vi "Seq Get Current Sequence.vi"(6 "config paths":T1, 8 "Error In":errorcluster, 9 "Segment Info In":T2, 10 "Basic Steps":string[](array[string]), 11 "VI Names":string[](array[string])) -> (0 "Error Out":errorcluster, 2 "Step Hisitory":string[](array[string]))   [LabVIEW 2018]
uses:
  type defs/Sequence Info.ctl
  type defs/config paths for seq def.ctl
panel:
  out "appended path":path
  out "file or folder exists?":bool
  out "File Name":string
  out "Add Step?":bool
  out "Segment Info Out":T2
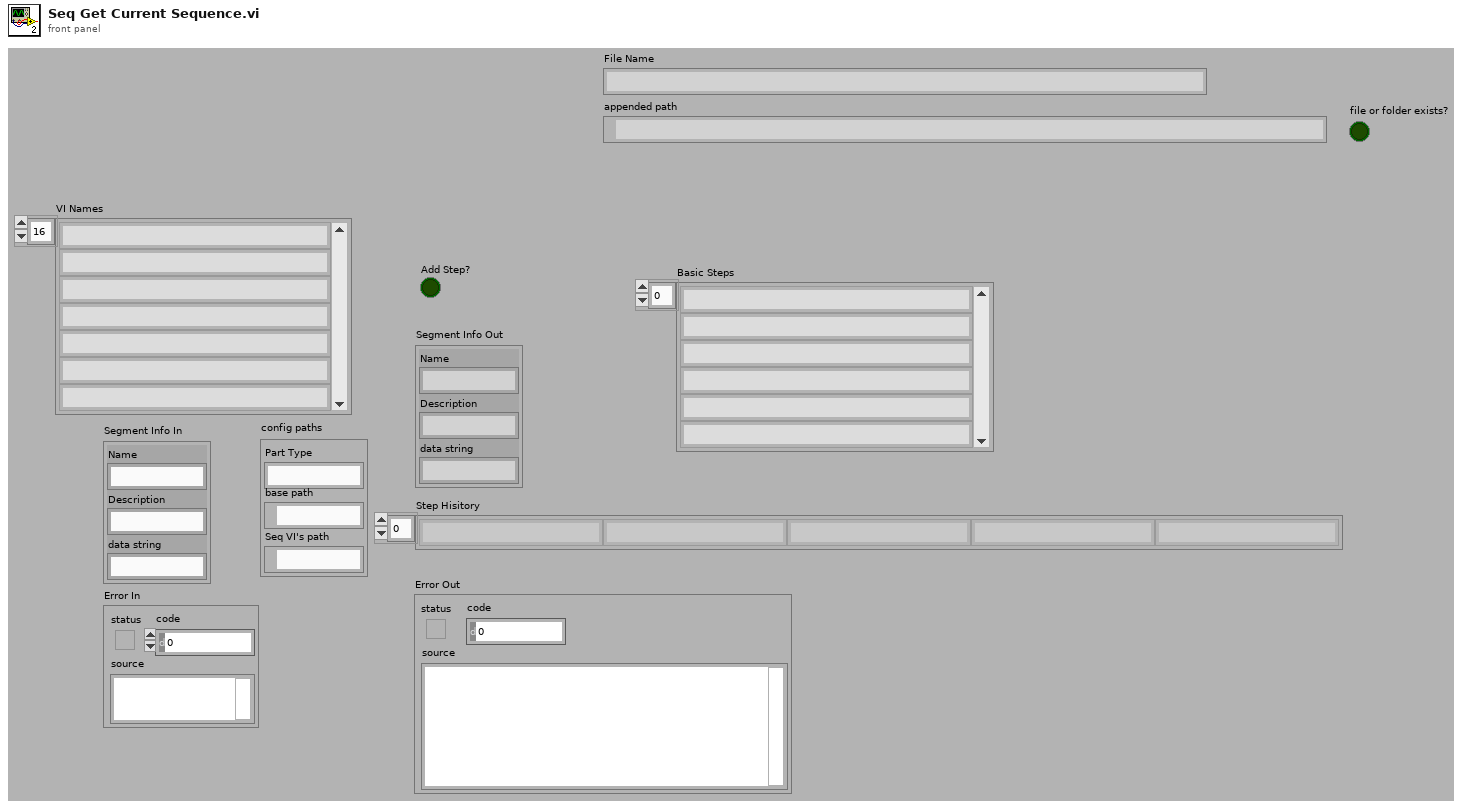
[diagram p1: front panel]
types:
  T1 = typedef "config paths for seq def.ctl" = cluster{"Part Type":string, "base path":path, "Seq VI's path":path}
  T2 = typedef "Sequence Info.ctl" = cluster{"Name":string, "Description":string, "data string":string}
  T3 = enum32{"Bad", "Idle", "Run top level", "Running"}
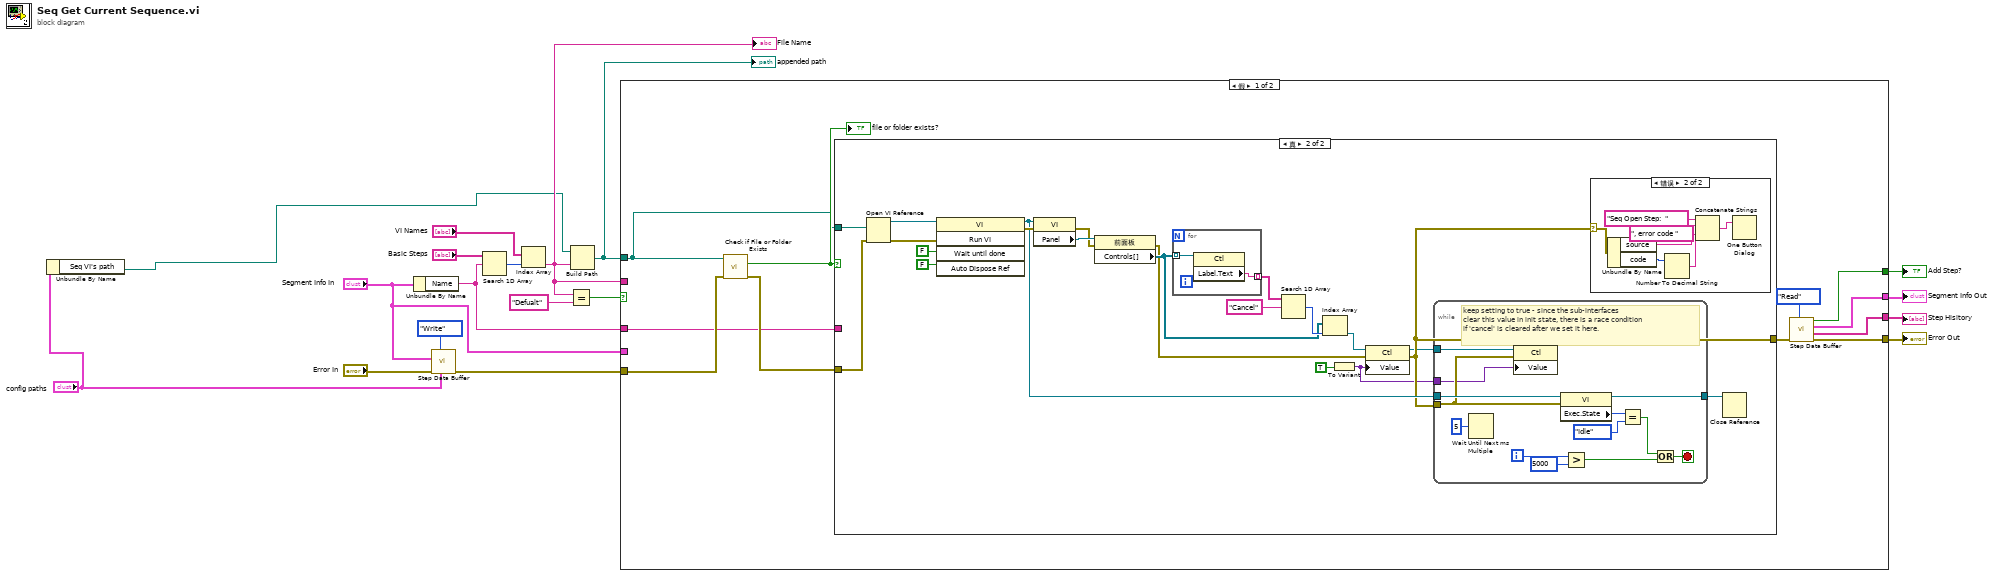
[diagram p0: block diagram]
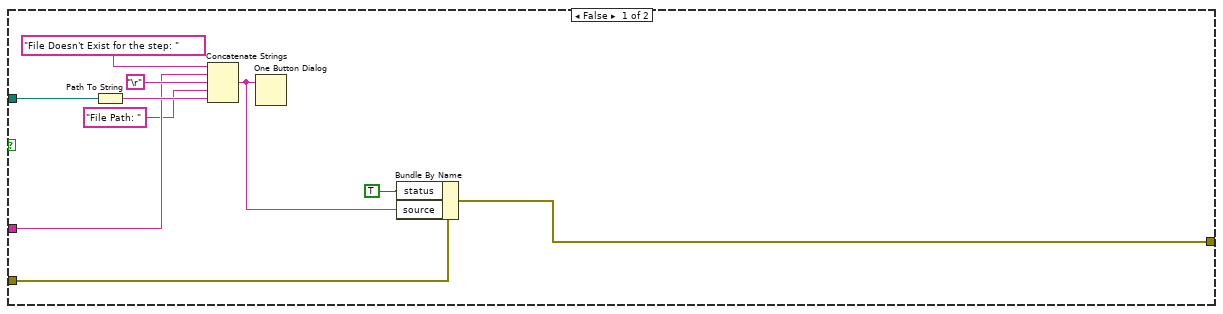
[diagram p2: hidden frame]
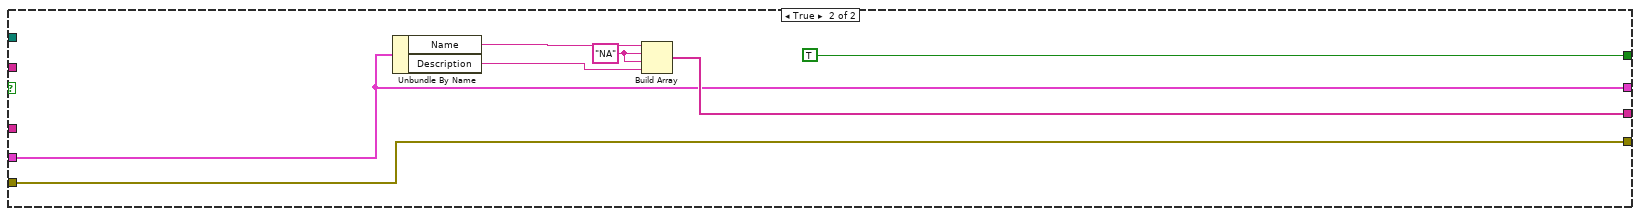
[diagram p4: hidden frame]
diagram:
  n1 = Unbundle By Name("config paths") -> ("Seq VI's path"=w1:path)
  n2 = Unbundle By Name("Segment Info In") -> ("Name"=w14:string)
  n3 = call "Step Data Buffer.vi"("config paths"="config paths", "Mode"=enum16{"Init", "Read", "Write"}."Write", "Error In"="Error In", "Segment Data"="Segment Info In") -> ("Error Out"=w11:errorcluster)  [unwired: 3 in, 4 out]
  n4 = Search 1D Array(1D array="Basic Steps", element=w14) -> (index of element=w10:i32)  [unwired: 1 in]
  n5 = Index Array(array="VI Names", index=w10) -> (element=w3:string)
  "File Name" <- w3
  n6 = Equal?(x=w3, y="Defualt") -> (x = y?=w8:bool)
  n7 = Build Path(base path=w1, name or relative path=w3) -> (appended path=w7:path)
  "appended path" <- w7
  n8 = case shown="假" w8 {
    tunnel: w7 -> [w28 _]
    tunnel: w11 -> [w27 w87]
    tunnel: [w23 w87] -> w15
    tunnel: w14 -> [w19 _]
    tunnel: [w22 w88] -> w18
    tunnel: [w20 TRUE ("Add Step?")] -> w6
    tunnel: "Segment Info In" -> [_ w85]
    tunnel: [w21 w85] -> w4
    tunnel: w3 -> [_ _]
    frame False {
      n9 = call <vilib>:"Check if File or Folder Exists.vi"("error in (no error)"=w27, "path"=w28) -> ("error out"=w26:errorcluster, "file or folder exists?"=w29:bool)  [unwired: 7 in, 1 out]
      "file or folder exists?" <- w29
      n10 = case shown="真" w29 {
        tunnel: w28 -> [w39 w60]
        tunnel: [w32 w46] -> w24
        tunnel: w26 -> [w33 w59]
        tunnel: w19 -> [w35 _]
        frame False {
          n11 = Path To String(path=w39) -> (string=w38:string)
          n12 = Concatenate Strings("File Doesn't Exist for the step: " ("string"), w35, "\r", "File Path: " ("string"), w38) -> (w31:string)
          n13 = One Button Dialog(message=w31) -> ()  [unwired: 1 in, 1 out]
          n14 = Bundle By Name(cluster=w33, "status"=TRUE, "source"=w31) -> (w32:errorcluster)
        }
        frame True {
          n15 = Open VI Reference(vi path=w60, error in (no error)=w59) -> (vi reference=w43:refnum<vi>, error out=w44:errorcluster)  [unwired: 4 in]
          n16 = invoke class="VI" method="Run VI"(reference=w43, error in=w44, "Wait until done"=FALSE ("Wait Until Done"), "Auto Dispose Ref"=FALSE ("Auto Dispose Reference")) -> (reference out=w47:refnum<vi>, error out=w49:errorcluster)  [unwired: 1 in, 3 out]
          n17 = property class="VI"(reference=w47, error in=w49) -> (error out=w50:errorcluster, "Panel"=w57:refnum<vi>)  [unwired: 1 out]
          n18 = property class="前面板"(reference=w57, error in=w50) -> (error out=w42:errorcluster, "Controls[]"=w53:refnum<vi>[])  [unwired: 1 out]
          n19 = for {
            tunnel: w53 -> [w75] mode=indexing
            tunnel: [w74] -> w56 mode=indexing
            n20 = property class="Ctl"(reference=w75) -> ("Label.Text"=w74:string)  [unwired: 1 in, 2 out]
          }
          n21 = Search 1D Array(1D array=w56, element="Cancel") -> (index of element=w54:i32)  [unwired: 1 in]
          n22 = Index Array(array=w53, index=w54) -> (element=w52:refnum<vi>)
          n23 = To Variant(anything=TRUE) -> (Variant=w40:variant)
          n24 = property class="Ctl"(reference=w52, error in=w42, "Value"=w40) -> (reference out=w41:refnum<vi>, error out=w46:errorcluster)
          n25 = while {
            tunnel: w47 -> [w73]
            tunnel: w46 -> [w62]
            tunnel: [w65] -> w45
            tunnel: w41 -> [w64]
            tunnel: w40 -> [w61]
            i -> [w68]
            stop <- w70 stop-if-true
            # "keep setting to true - since the sub-interfaces\nclear this value in init state, there is a race condition\nif 'cancel' is cleared after we set it here."
            n26 = Wait Until Next ms Multiple(millisecond multiple=u32 5) -> ()  [unwired: 1 out]
            n27 = property class="Ctl"(reference=w64, error in=w62, "Value"=w61) -> ()  [unwired: 2 out]
            n28 = property class="VI"(reference=w73, error in=w62) -> (reference out=w65:refnum<vi>, "Exec.State"=w72:T3)  [unwired: 1 out]
            n29 = Greater?(x=w68, y=5000) -> (0:w66:bool)
            n30 = Equal?(x=w72, y=T3."Idle") -> (x = y?=w69:bool)
            n31 = Or(x=w69, y=w66) -> (x .or. y?=w70:bool)
          }
          n32 = case shown="错误" w46 {
            selector: w46 -> [_ w81]
            frame No Error {
            }
            frame Error {
              n33 = Unbundle By Name(w81) -> ("source"=w79:string, "code"=w77:i32)
              n34 = Number To Decimal String(number=w77) -> (decimal integer string=w76:string)  [unwired: 1 in]
              n35 = Concatenate Strings("Seq Open Step:  " ("message"), w79, ", error code " ("string"), w76) -> (w80:string)
              n36 = One Button Dialog(message=w80) -> ()  [unwired: 1 in, 1 out]
            }
          }
          n37 = Close Reference(reference=w45) -> ()  [unwired: 1 in, 1 out]
        }
      }
      n38 = call "Step Data Buffer.vi"("Mode"=enum16{"Init", "Read", "Write"}."Read", "Error In"=w24) -> ("Error Out"=w23:errorcluster, "Step Hisitory Out"=w22:string[], "Segment Data"=w21:T2, "Add Step? Out"=w20:bool)  [unwired: 5 in, 1 out]
    }
    frame True {
      w89 = "NA" ("element")
      n39 = Unbundle By Name(w85) -> ("Name"=w84:string, "Description"=w83:string)
      n40 = Build Array(w84, w89, w89, w83) -> (w88:string[])
    }
  }
  "Step Hisitory" <- w18
  "Segment Info Out" <- w4
  "Add Step?" <- w6
  "Error Out" <- w15
